vi "classes.vi"(0 "HGF_DFSMFactory":refnum<class "HGF_DFSMFactory.lvclass">, 1 "className":string, 5 "error in (no error)":errorcluster) -> (14 "HGF_DFSMFactory dup":refnum<class "HGF_DFSMFactory.lvclass">, 16 "Object":refnum<class>, 19 "error out":errorcluster)   [LabVIEW 2012, in "HGF_DeviceFSM.lvlib" / "HGF_DFSMFactory.lvclass"]
doc: "This dynamaic dispatch VI contains constant objects of all classes that can be produced by HGF_Factory.\nClass has to be defined by name. \n\nOptionally, you can also specifiy a Class Path String instead, but you have to make sure that all dependencies are available.\n\nChild classes have to override it to define additional classes."
uses:
  HGF_DFSMFactory.lvclass
  HGF_DFSMVisitor/HGF_DFSMVisitor.lvclass
  HGF_TaskDFSM/HGF_TaskDFSM.lvclass
  HGF_BaseClasses/HGF_Factory/HGF_Factory.lvclass
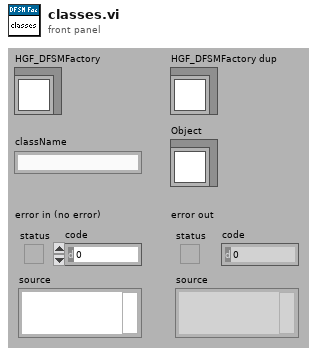
[diagram p1: front panel]
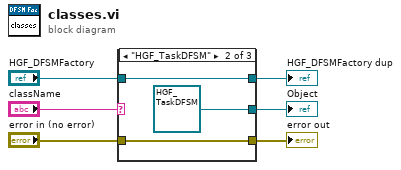
[diagram p0: block diagram]
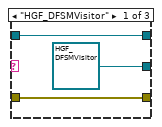
[diagram p2: hidden frame]
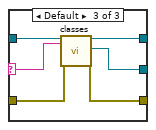
[diagram p3: hidden frame]
diagram:
  n1 = case shown="\"HGF_TaskDFSM\"" "className" {
    selector: "className" -> [_ _ w13]
    tunnel: "HGF_DFSMFactory" -> [w8 w11 w18]
    tunnel: "error in (no error)" -> [w7 w10 w17]
    tunnel: [w8 w11 w16] -> w4
    tunnel: [refnum<class "HGF_DFSMVisitor.lvclass"> refnum ("HGF_DeviceFSM.lvlib:HGF_DFSMVisitor.lvclass") refnum<class "HGF_TaskDFSM.lvclass"> refnum ("HGF_DeviceFSM.lvlib:HGF_TaskDFSM.lvclass") w15] -> w3
    tunnel: [w7 w10 w14] -> w2
    frame "HGF_DFSMVisitor" {
    }
    frame "HGF_TaskDFSM" {
    }
    frame Default {
      n2 = call-parent "classes.vi"("HGF_Factory"=w18, "className"=w13, "error in (no error)"=w17) -> ("HGF_Factory dup"=w16:refnum<class "HGF_DFSMFactory.lvclass">, "Object"=w15:refnum<class>, "error out"=w14:errorcluster)  [unwired: 14 out]
    }
  }
  "error out" <- w2
  "HGF_DFSMFactory dup" <- w4
  "Object" <- w3
